vi "Write Standard.vi"(8 "error in (no error)":errorcluster, 10 "Standard":string, 11 "Harmonics_Relative_Power in":refnum<class "Harmonics_Relative_Power.lvclass">) -> (0 "error out":errorcluster, 3 "Harmonics_Relative_Power out":refnum<class "Harmonics_Relative_Power.lvclass">)   [LabVIEW 2018, in "SeqAuto Evaluations.lvlib" / "Harmonics_Relative_Power.lvclass"]
uses:
  Harmonics_Relative_Power.lvclass
  Harmonics_Relative_Power.lvclass/Harmonics_Relative_Power.ctl
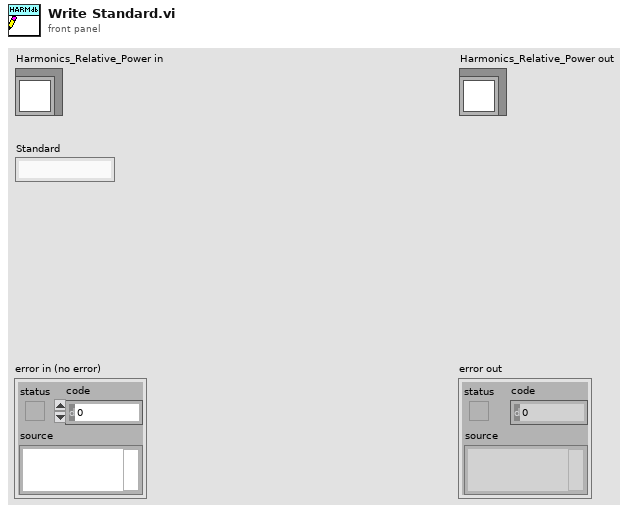
[diagram p1: front panel]
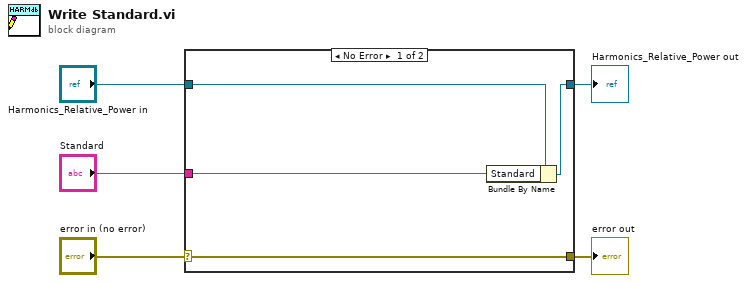
[diagram p0: block diagram]
diagram:
  n1 = case shown="No Error" "error in (no error)" {
    selector: "error in (no error)" -> [w9 w10]
    tunnel: [w9 w10] -> w4
    tunnel: [w7 w11] -> w2
    tunnel: "Harmonics_Relative_Power in" -> [w8 w11]
    tunnel: "Standard" -> [w6 _]
    frame No Error {
      n2 = Bundle By Name(cluster=w8, "Standard"=w6) -> (w7:refnum<class "Harmonics_Relative_Power.lvclass">)
    }
    frame Error {
    }
  }
  "error out" <- w4
  "Harmonics_Relative_Power out" <- w2
